vi "Get mouse coordinates.vi"(8 "error in":errorcluster) -> (0 "error out":errorcluster, 3 "axis info":T1)   [LabVIEW 2020]
uses:
  <vilib>/Utility/inputDevices.llb/mouseAcquire.vi
  <vilib>/Utility/inputDevices.llb/closeMouse.vi
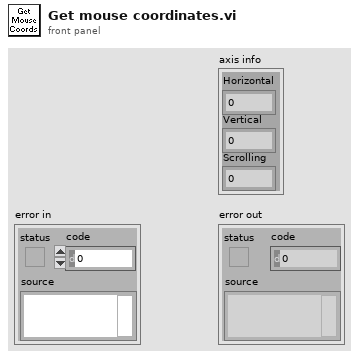
[diagram p1: front panel]
types:
  T1 = cluster{"Horizontal":i32, "Vertical":i32, "Scrolling":i32}
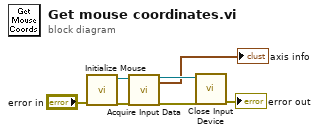
[diagram p0: block diagram]
diagram:
  n1 = call <vilib>:"Initialize Mouse.vi"("error in (no error)"="error in") -> ("error out"=w4:errorcluster, "device ID"=w6:refnum<k1>)  [unwired: 9 in]
  n2 = call-poly <vilib>:"Acquire Input Data.vi"("device ID"=w6, "error in (no error)"=w4) -> ("device ID"=w7:refnum<k1>, "axis info"=→"axis info":T1, "error out"=w5:errorcluster)  [unwired: 14 in, 1 out]
  n3 = call-poly <vilib>:"Close Input Device.vi"("error in (no error)"=w5, "device ID"=w7) -> ("error out"=→"error out":errorcluster)  [unwired: 8 in]
